vi "Front End.vi"() -> ()   [LabVIEW 2014]
uses:
  <vilib>/Utility/file.llb/Write To Spreadsheet File (DBL).vi
  <vilib>/Utility/file.llb/Write To Spreadsheet File (string).vi
  <vilib>/Utility/file.llb/Read From Spreadsheet File (DBL).vi
panel:
  in  "WebBrowser":refnum<k7>(container)
  in  "Tab Control":enum32{"Display", "Config"}(tab)
  in  "Control":enum32{"Auto", "Manual"}(tab)
  in  "Auto Stop":bool
  in  "Manual Stop":bool
  in  "Record Button":bool
  in  "Manual Throttle":dbl
  out "RPM":dbl
  out "Battery Life (h)":dbl
  out "Torque":dbl
  out "Horsepower":dbl
  in  "Main Stop":bool
  out "Flowrate":dbl
  out "Total Fuel":dbl
  out "Total Fuel Graph":cluster{u32, dbl}[](graph)
  out "Throttle":dbl
  in  "Time Unit":u16(ring)=1 items=["ms", "s"]
  in  "Control File":path
  in  "DAQ Device Name":tag="cDAQ1Mod1"
  in  "Output Directory":path
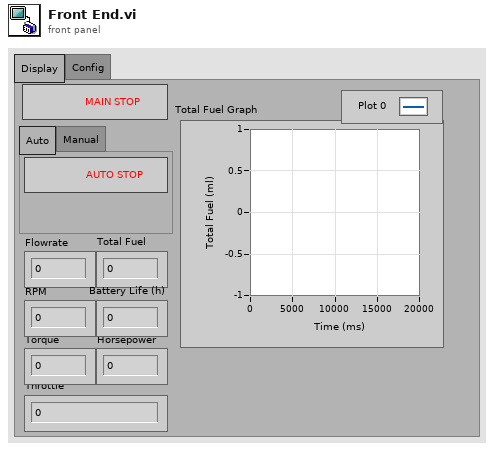
[diagram p1: front panel]
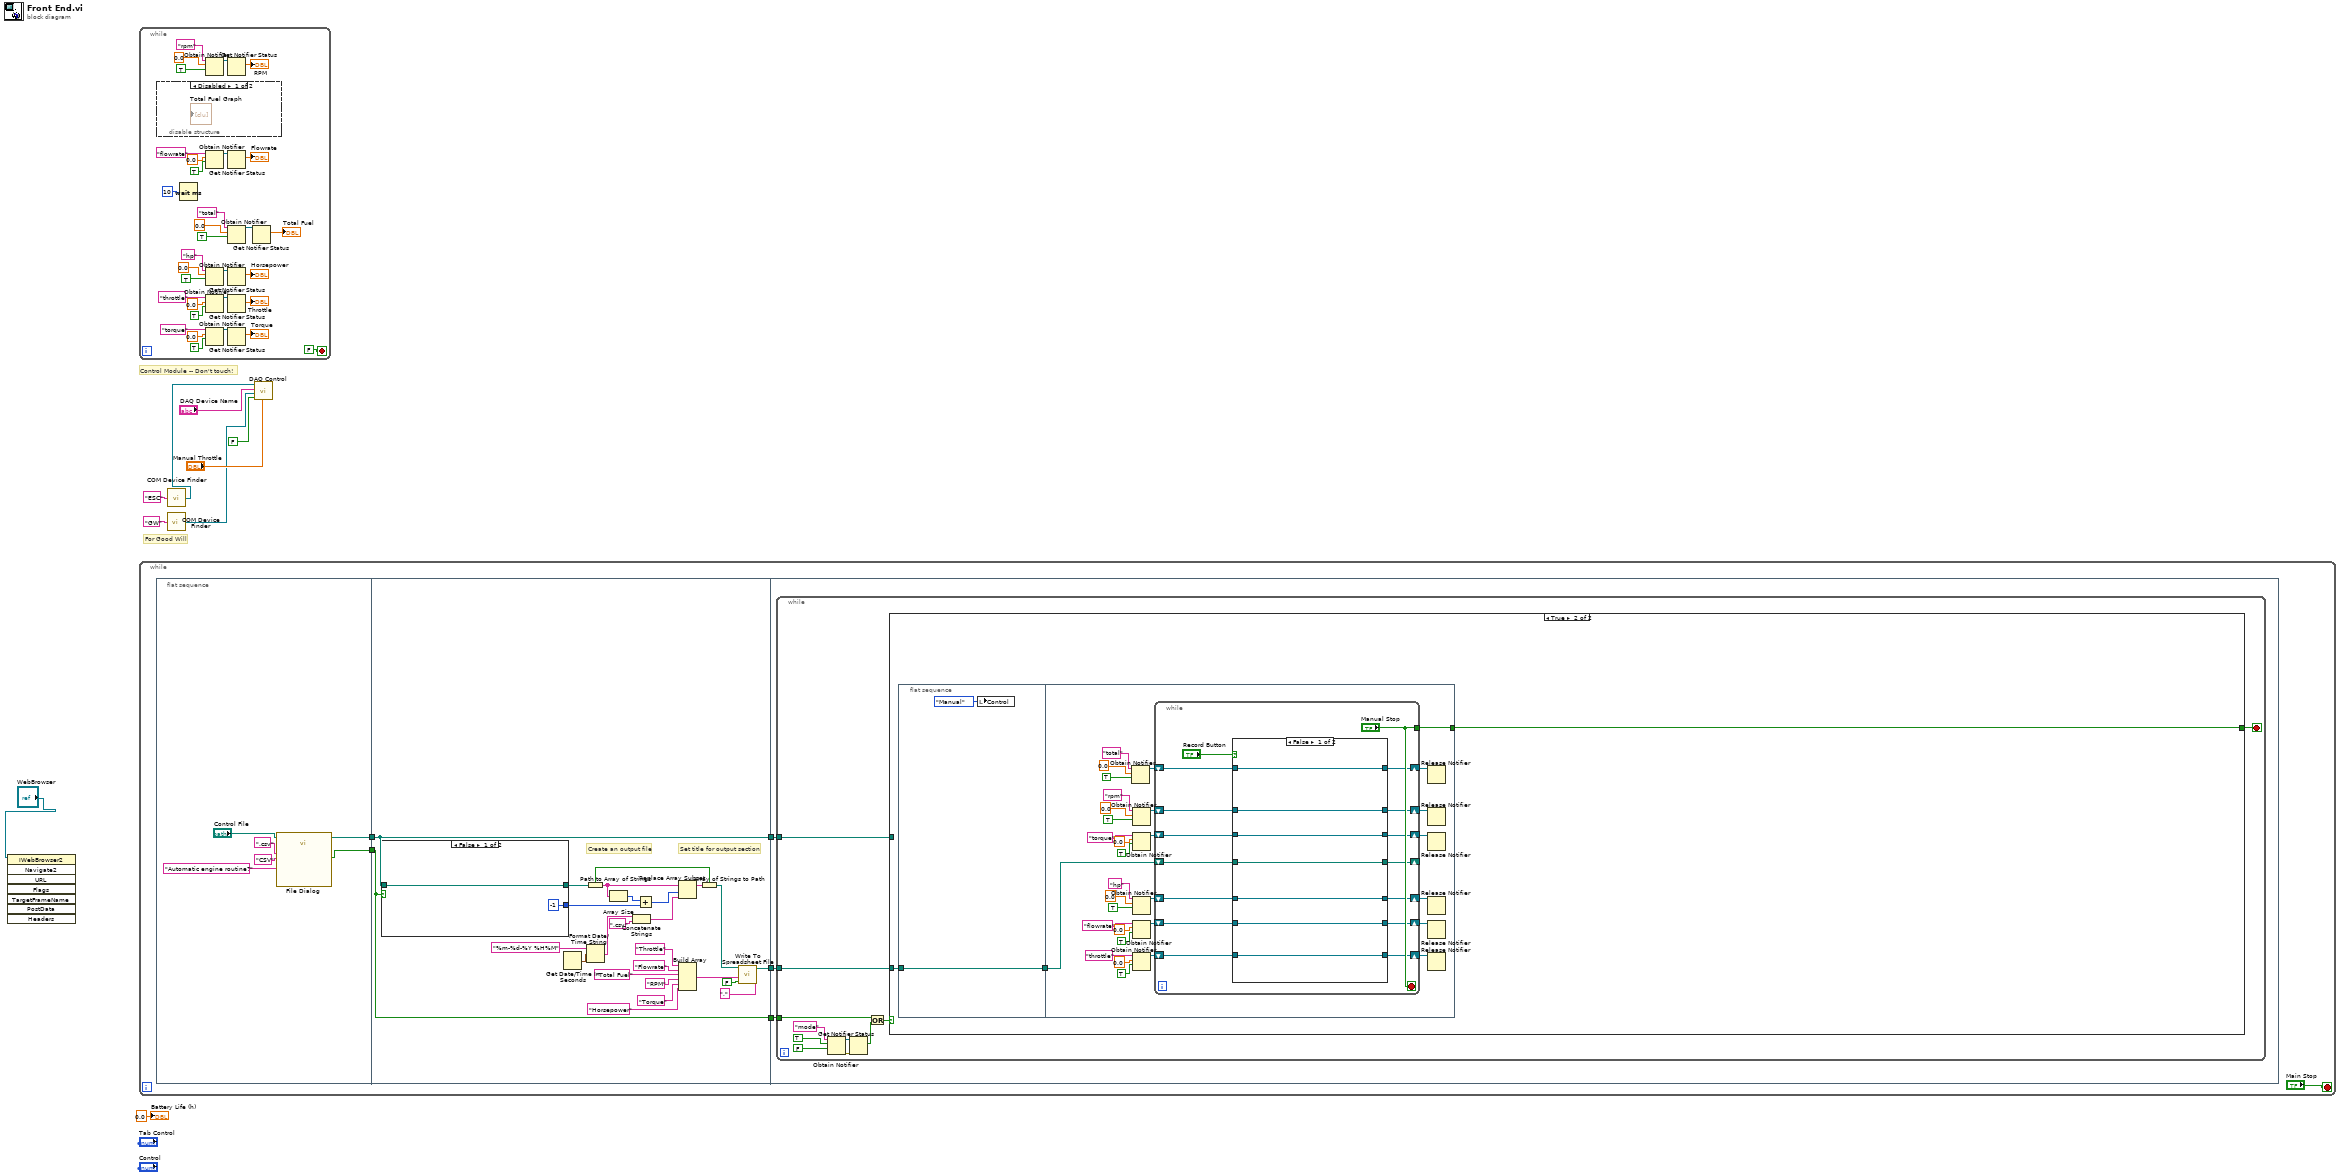
[diagram p0: block diagram]
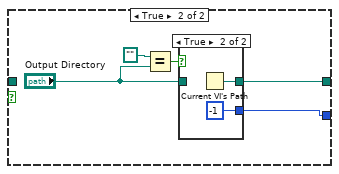
[diagram p3: hidden frame]
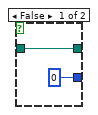
[diagram p4: hidden frame]
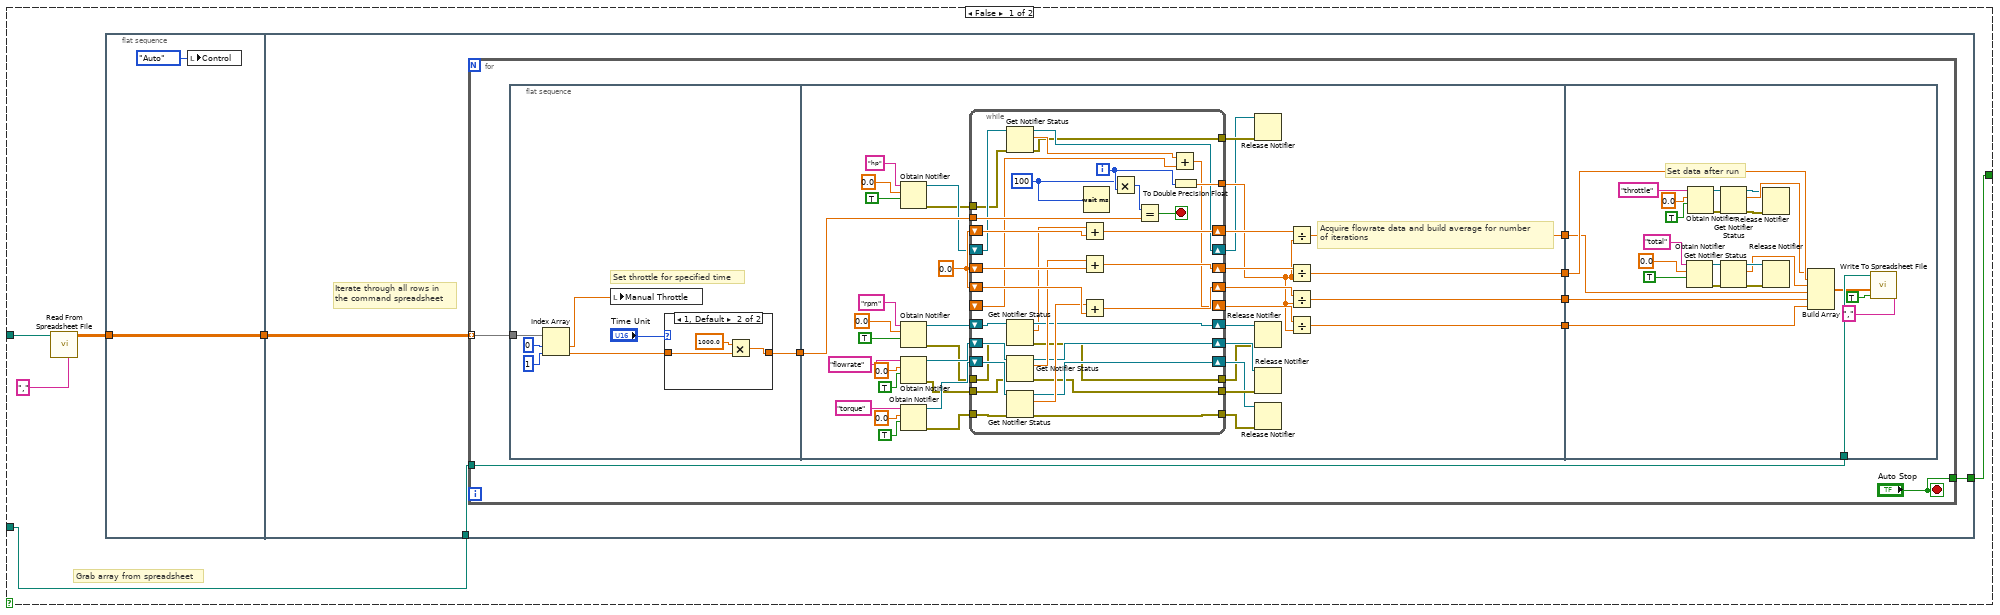
[diagram p5: hidden frame]
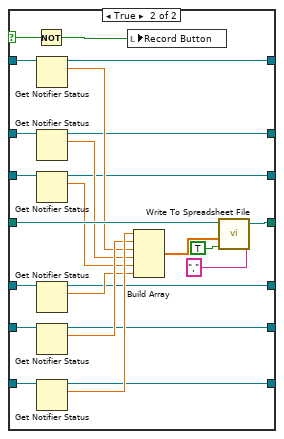
[diagram p7: hidden frame]
diagram:
  # "For Good Will"
  # "Control Module -- Don't touch!"
  n1 = invoke class="IWebBrowser2" method="Navigate2"(reference="WebBrowser") -> ()  [unwired: 7 in, 8 out]
  n2 = while {
    stop <- FALSE stop-if-true
    n3 = disable-structure shown="Disabled" {
      frame Disabled {
      }
      frame Enabled {
      }
    }
    n4 = Wait (ms)(milliseconds to wait=u32 10) -> ()  [unwired: 1 out]
    n5 = Obtain Notifier(name (unnamed)="rpm", notification data type=0.0, create if not found? (T)=TRUE) -> (notifier out=w21:refnum<notifier>)  [unwired: 1 in, 2 out]
    n6 = Obtain Notifier(name (unnamed)="flowrate", notification data type=0.0, create if not found? (T)=TRUE) -> (notifier out=w19:refnum<notifier>)  [unwired: 1 in, 2 out]
    n7 = Obtain Notifier(name (unnamed)="hp", notification data type=0.0, create if not found? (T)=TRUE) -> (notifier out=w20:refnum<notifier>)  [unwired: 1 in, 2 out]
    n8 = Obtain Notifier(name (unnamed)="throttle", notification data type=0.0, create if not found? (T)=TRUE) -> (notifier out=w18:refnum<notifier>)  [unwired: 1 in, 2 out]
    n9 = Obtain Notifier(name (unnamed)="torque", notification data type=0.0, create if not found? (T)=TRUE) -> (notifier out=w23:refnum<notifier>)  [unwired: 1 in, 2 out]
    n10 = Obtain Notifier(name (unnamed)="total", notification data type=0.0, create if not found? (T)=TRUE) -> (notifier out=w22:refnum<notifier>)  [unwired: 1 in, 2 out]
    n11 = Get Notifier Status(notifier=w21) -> (current notification=→"RPM":dbl)  [unwired: 1 in, 4 out]
    n12 = Get Notifier Status(notifier=w19) -> (current notification=→"Flowrate":dbl)  [unwired: 1 in, 4 out]
    n13 = Get Notifier Status(notifier=w20) -> (current notification=→"Horsepower":dbl)  [unwired: 1 in, 4 out]
    n14 = Get Notifier Status(notifier=w18) -> (current notification=→"Throttle":dbl)  [unwired: 1 in, 4 out]
    n15 = Get Notifier Status(notifier=w23) -> (current notification=→"Torque":dbl)  [unwired: 1 in, 4 out]
    n16 = Get Notifier Status(notifier=w22) -> (current notification=→"Total Fuel":dbl)  [unwired: 1 in, 4 out]
  }
  n17 = while {
    stop <- "Main Stop" stop-if-true
    n18 = flat-sequence {
      tunnel: [w53] -> w47
      tunnel: [w51] -> w46
      tunnel: [w72] -> w45
      tunnel: [w59] -> w44
      tunnel: w47 -> [w59]
      tunnel: [w56] -> w43
      tunnel: w46 -> [w56]
      tunnel: w45 -> [w92]
      tunnel: w44 -> [w91]
      tunnel: w43 -> [w90]
      frame #0 {
        n19 = call "File Dialog"("start path"="Control File", "prompt"="Automatic engine routine?", "pattern (all files)"=".csv", "pattern label"="CSV") -> ("selected path"=w53:path, "cancelled"=w51:bool)  [unwired: 8 in, 2 out]
      }
      frame #1 {
        # "Create an output file"
        # "Set title for output section"
        n20 = case shown="False" w56 {
          tunnel: w59 -> [w80 _]
          tunnel: [w80 w85] -> w58
          tunnel: [-1 w81] -> w54
          frame False {
          }
          frame True {
            n21 = Equal?(x=path "", y="Output Directory") -> (x = y?=w84:bool)
            n22 = case shown="True" w84 {
              tunnel: [w87 w89] -> w85
              tunnel: "Output Directory" -> [w87 _]
              tunnel: [0 -1] -> w81
              frame False {
              }
              frame True {
                n23 = Current VI's Path() -> (path=w89:path)
              }
            }
          }
        }
        n24 = Get Date/Time In Seconds() -> (seconds since 1Jan1904=w69:timestamp)
        n25 = Path to Array of Strings(0:w58) -> (1:w64:bool, 2:w71:string[])
        n26 = Format Date/Time String(time format string (%c)="%m-%d-%Y %H%M", seconds (now)=w69) -> (date/time string=w68:string)  [unwired: 1 in]
        n27 = Array Size(array=w71) -> (size(s)=w55:i32)
        n28 = Concatenate Strings(w68, ".csv") -> (w66:string)
        n29 = Add(x=w55, y=w54) -> (x+y=w70:i32)
        n30 = Replace Array Subset(array=w71, new element=w66, index=w70) -> (w65:string[])
        n31 = Build Array("Throttle" ("element"), "Flowrate", "Total Fuel" ("element"), "RPM" ("element"), "Torque" ("element"), "Horsepower" ("element")) -> (w74:string[])
        n32 = Array of Strings to Path(0:w65, 1:w64) -> (2:w63:path)
        n33 = call-poly <vilib>:"Write To Spreadsheet File.vi"("delimiter (\\t)"="," ("delimiter (\\t)"), "append to file? (new file:F)"=FALSE, "1D data"=w74, "file path (dialog if empty)"=w63) -> ("new file path (Not A Path if cancelled)"=w72:path)  [unwired: 4 in]
      }
      frame #2 {
        n34 = while {
          tunnel: w92 -> [w103]
          tunnel: w91 -> [w102]
          tunnel: w90 -> [w95]
          stop <- w93 stop-if-true
          n35 = Obtain Notifier(name (unnamed)="mode", notification data type=TRUE, create if not found? (T)=FALSE) -> (notifier out=w101:refnum<notifier>, error out=w98:errorcluster)  [unwired: 1 in, 1 out]
          n36 = Get Notifier Status(notifier=w101, error in (no error)=w98) -> (current notification=w96:bool)  [unwired: 4 out]
          n37 = Or(x=w95, y=w96) -> (x .or. y?=w94:bool)
          n38 = case shown="True" w94 {
            tunnel: w103 -> [w107 w233]
            tunnel: w102 -> [w106 _]
            tunnel: [w104 w231] -> w93
            frame False {
              # "Grab array from spreadsheet"
              n39 = call-poly <vilib>:"Read From Spreadsheet File.vi"("delimiter (\\t)"="," ("delimiter (\\t)"), "file path (dialog if empty)"=w106) -> ("all rows"=w109:dbl[][])  [unwired: 5 in, 4 out]
              n40 = flat-sequence {
                tunnel: w109 -> [w111]
                tunnel: [w111] -> w105
                tunnel: w107 -> [w113]
                tunnel: w105 -> [w114]
                tunnel: [w112] -> w104
                frame #0 {
                  n41 = local write "Control"(enum32{"Auto", "Manual"}."Auto" ("Control")) -> ()
                }
                frame #1 {
                  # "Iterate through all rows in \nthe command spreadsheet"
                  n42 = for {
                    tunnel: w114 -> [w122] mode=indexing
                    tunnel: w113 -> [w120]
                    tunnel: ["Auto Stop"] -> w112
                    stop <- "Auto Stop" stop-if-true
                    n43 = flat-sequence {
                      tunnel: w122 -> [w129]
                      tunnel: [w124] -> w121
                      tunnel: w121 -> [w172]
                      tunnel: [w165] -> w119
                      tunnel: [w164] -> w118
                      tunnel: [w163] -> w117
                      tunnel: [w162] -> w116
                      tunnel: w120 -> [w229]
                      tunnel: w119 -> [w227]
                      tunnel: w118 -> [w226]
                      tunnel: w117 -> [w225]
                      tunnel: w116 -> [w224]
                      frame #0 {
                        # "Set throttle for specified time"
                        n44 = Index Array(array=w129, index #1=0 ("index"), index #2=1 ("index")) -> (element #1=w123:dbl, element #2=w125:dbl)
                        n45 = local write "Manual Throttle"(w123) -> ()
                        n46 = case shown="1, Default" "Time Unit" {
                          tunnel: w125 -> [w130 w133]
                          tunnel: [w130 w131] -> w124
                          frame 0 {
                          }
                          frame 1, Default {
                            n47 = Multiply(x=1000.0, y=w133) -> (x*y=w131:dbl)
                          }
                        }
                      }
                      frame #1 {
                        w171 = 0.0
                        # "Acquire flowrate data and build average for number\nof iterations"
                        n48 = Obtain Notifier(name (unnamed)="hp", notification data type=0.0, create if not found? (T)=TRUE) -> (notifier out=w149:refnum<notifier>, error out=w136:errorcluster)  [unwired: 1 in, 1 out]
                        n49 = Obtain Notifier(name (unnamed)="rpm", notification data type=0.0, create if not found? (T)=TRUE) -> (notifier out=w146:refnum<notifier>, error out=w137:errorcluster)  [unwired: 1 in, 1 out]
                        n50 = Obtain Notifier(name (unnamed)="flowrate", notification data type=0.0, create if not found? (T)=TRUE) -> (notifier out=w148:refnum<notifier>, error out=w144:errorcluster)  [unwired: 1 in, 1 out]
                        n51 = Obtain Notifier(name (unnamed)="torque", notification data type=0.0, create if not found? (T)=TRUE) -> (notifier out=w147:refnum<notifier>, error out=w140:errorcluster)  [unwired: 1 in, 1 out]
                        n52 = while {
                          shift-right: [w195] -> w167
                          shift-left: w171 -> [w196]
                          tunnel: w172 -> [w206]
                          tunnel: [w201] -> w166
                          shift-right: [w199] -> w170
                          shift-left: w171 -> [w200]
                          shift-right: [w197] -> w169
                          shift-left: w171 -> [w198]
                          shift-right: [w194] -> w168
                          shift-left: _ -> [w193]
                          shift-right: [w190] -> w134
                          shift-left: w149 -> [w191]
                          shift-right: [w185] -> w145
                          shift-left: w148 -> [w189]
                          shift-right: [w184] -> w142
                          shift-left: w147 -> [w187]
                          shift-right: [w182] -> w139
                          shift-left: w146 -> [w183]
                          tunnel: w144 -> [w180]
                          tunnel: [w179] -> w143
                          tunnel: [w178] -> w141
                          tunnel: w140 -> [w177]
                          tunnel: [w176] -> w138
                          tunnel: w137 -> [w175]
                          tunnel: w136 -> [w174]
                          tunnel: [w173] -> w135
                          i -> [w204]
                          stop <- w205 stop-if-true
                          w203 = u32 100 ("milliseconds to wait")
                          n53 = Get Notifier Status(notifier=w191, error in (no error)=w174) -> (notifier out=w190:refnum<notifier>, current notification=w192:dbl, error out=w173:errorcluster)  [unwired: 2 out]
                          n54 = Get Notifier Status(notifier=w183, error in (no error)=w175) -> (notifier out=w182:refnum<notifier>, current notification=w181:dbl, error out=w176:errorcluster)  [unwired: 2 out]
                          n55 = Get Notifier Status(notifier=w189, error in (no error)=w180) -> (notifier out=w185:refnum<notifier>, current notification=w188:dbl, error out=w179:errorcluster)  [unwired: 2 out]
                          n56 = Get Notifier Status(notifier=w187, error in (no error)=w177) -> (notifier out=w184:refnum<notifier>, current notification=w186:dbl, error out=w178:errorcluster)  [unwired: 2 out]
                          n57 = Add(x=w181, y=w198) -> (x+y=w197:dbl)
                          n58 = Add(x=w188, y=w200) -> (x+y=w199:dbl)
                          n59 = Add(x=w186, y=w196) -> (x+y=w195:dbl)
                          n60 = Wait (ms)(milliseconds to wait=w203) -> ()  [unwired: 1 out]
                          n61 = Multiply(x=w203, y=w204) -> (x*y=w202:u32)
                          n62 = Equal?(x=w202, y=w206) -> (x = y?=w205:bool)
                          n63 = Add(x=w192, y=w193) -> (x+y=w194:dbl)
                          n64 = To Double Precision Float(number=w204) -> (double precision float=w201:dbl)
                        }
                        n65 = Release Notifier(notifier=w134, error in (no error)=w135) -> ()  [unwired: 1 in, 3 out]
                        n66 = Release Notifier(notifier=w139, error in (no error)=w138) -> ()  [unwired: 1 in, 3 out]
                        n67 = Release Notifier(notifier=w145, error in (no error)=w143) -> ()  [unwired: 1 in, 3 out]
                        n68 = Release Notifier(notifier=w142, error in (no error)=w141) -> ()  [unwired: 1 in, 3 out]
                        n69 = Divide(x=w169, y=w166) -> (x/y=w164:dbl)
                        n70 = Divide(x=w170, y=w166) -> (x/y=w165:dbl)
                        n71 = Divide(x=w167, y=w166) -> (x/y=w163:dbl)
                        n72 = Divide(x=w168, y=w166) -> (x/y=w162:dbl)
                      }
                      frame #2 {
                        # "Set data after run"
                        n73 = Obtain Notifier(name (unnamed)="total", notification data type=0.0, create if not found? (T)=TRUE) -> (notifier out=w214:refnum<notifier>, error out=w209:errorcluster)  [unwired: 1 in, 1 out]
                        n74 = Obtain Notifier(name (unnamed)="throttle", notification data type=0.0, create if not found? (T)=TRUE) -> (notifier out=w222:refnum<notifier>, error out=w216:errorcluster)  [unwired: 1 in, 1 out]
                        n75 = Get Notifier Status(notifier=w222, error in (no error)=w216) -> (notifier out=w217:refnum<notifier>, current notification=w218:dbl, error out=w215:errorcluster)  [unwired: 2 out]
                        n76 = Get Notifier Status(notifier=w214, error in (no error)=w209) -> (notifier out=w210:refnum<notifier>, current notification=w207:dbl, error out=w208:errorcluster)  [unwired: 2 out]
                        n77 = Release Notifier(notifier=w217, error in (no error)=w215) -> ()  [unwired: 1 in, 3 out]
                        n78 = Release Notifier(notifier=w210, error in (no error)=w208) -> ()  [unwired: 1 in, 3 out]
                        n79 = Build Array(w218, w227, w207, w226, w225, w224) -> (w223:dbl[])
                        n80 = call-poly <vilib>:"Write To Spreadsheet File.vi"("delimiter (\\t)"="," ("delimiter (\\t)"), "append to file? (new file:F)"=TRUE, "1D data"=w223, "file path (dialog if empty)"=w229) -> ()  [unwired: 4 in, 1 out]
                      }
                    }
                  }
                }
              }
            }
            frame True {
              n81 = flat-sequence {
                tunnel: w233 -> [w235]
                tunnel: [w235] -> w232
                tunnel: w232 -> [w267]
                tunnel: [w266] -> w231
                frame #0 {
                  n82 = local write "Control"(enum32{"Auto", "Manual"}."Manual" ("Tab Control 2")) -> ()
                }
                frame #1 {
                  n83 = Obtain Notifier(name (unnamed)="total", notification data type=0.0, create if not found? (T)=TRUE) -> (notifier out=w245:refnum<notifier>)  [unwired: 1 in, 2 out]
                  n84 = Obtain Notifier(name (unnamed)="rpm", notification data type=0.0, create if not found? (T)=TRUE) -> (notifier out=w244:refnum<notifier>)  [unwired: 1 in, 2 out]
                  n85 = Obtain Notifier(name (unnamed)="torque", notification data type=0.0, create if not found? (T)=TRUE) -> (notifier out=w243:refnum<notifier>)  [unwired: 1 in, 2 out]
                  n86 = Obtain Notifier(name (unnamed)="hp", notification data type=0.0, create if not found? (T)=TRUE) -> (notifier out=w242:refnum<notifier>)  [unwired: 1 in, 2 out]
                  n87 = Obtain Notifier(name (unnamed)="flowrate", notification data type=0.0, create if not found? (T)=TRUE) -> (notifier out=w246:refnum<notifier>)  [unwired: 1 in, 2 out]
                  n88 = Obtain Notifier(name (unnamed)="throttle", notification data type=0.0, create if not found? (T)=TRUE) -> (notifier out=w247:refnum<notifier>)  [unwired: 1 in, 2 out]
                  n89 = while {
                    tunnel: ["Manual Stop"] -> w266
                    shift-right: [w268] -> _
                    shift-left: w267 -> [w282]
                    shift-right: [w270] -> w237
                    shift-left: w246 -> [w279]
                    shift-right: [w273] -> w240
                    shift-left: w245 -> [w278]
                    shift-right: [w269] -> w236
                    shift-left: w247 -> [w280]
                    shift-right: [w274] -> w241
                    shift-left: w243 -> [w276]
                    shift-right: [w272] -> w239
                    shift-left: w244 -> [w277]
                    shift-right: [w271] -> w238
                    shift-left: w242 -> [w275]
                    stop <- "Manual Stop" stop-if-true
                    n90 = case shown="False" "Record Button" {
                      selector: "Record Button" -> [_ w315]
                      tunnel: w282 -> [w284 w313]
                      tunnel: w280 -> [w285 w309]
                      tunnel: w279 -> [w286 w307]
                      tunnel: w278 -> [w289 w305]
                      tunnel: w277 -> [w288 w303]
                      tunnel: w276 -> [w290 w301]
                      tunnel: w275 -> [w287 w299]
                      tunnel: [w290 w297] -> w274
                      tunnel: [w289 w296] -> w273
                      tunnel: [w288 w295] -> w272
                      tunnel: [w287 w294] -> w271
                      tunnel: [w286 w293] -> w270
                      tunnel: [w285 w292] -> w269
                      tunnel: [w284 w291] -> w268
                      frame False {
                      }
                      frame True {
                        n91 = Not(x=w315) -> (.not. x?=w314:bool)
                        n92 = Get Notifier Status(notifier=w305) -> (notifier out=w296:refnum<notifier>, current notification=w304:dbl)  [unwired: 1 in, 3 out]
                        n93 = Get Notifier Status(notifier=w303) -> (notifier out=w295:refnum<notifier>, current notification=w302:dbl)  [unwired: 1 in, 3 out]
                        n94 = Get Notifier Status(notifier=w301) -> (notifier out=w297:refnum<notifier>, current notification=w300:dbl)  [unwired: 1 in, 3 out]
                        n95 = Get Notifier Status(notifier=w299) -> (notifier out=w294:refnum<notifier>, current notification=w298:dbl)  [unwired: 1 in, 3 out]
                        n96 = Get Notifier Status(notifier=w307) -> (notifier out=w293:refnum<notifier>, current notification=w306:dbl)  [unwired: 1 in, 3 out]
                        n97 = Get Notifier Status(notifier=w309) -> (notifier out=w292:refnum<notifier>, current notification=w308:dbl)  [unwired: 1 in, 3 out]
                        n98 = local write "Record Button"(w314) -> ()
                        n99 = Build Array(w308, w306, w304, w302, w300, w298) -> (w312:dbl[])
                        n100 = call-poly <vilib>:"Write To Spreadsheet File.vi"("delimiter (\\t)"="," ("delimiter (\\t)"), "append to file? (new file:F)"=TRUE, "1D data"=w312, "file path (dialog if empty)"=w313) -> ("new file path (Not A Path if cancelled)"=w291:path)  [unwired: 4 in]
                      }
                    }
                  }
                  n101 = Release Notifier(notifier=w240) -> ()  [unwired: 2 in, 3 out]
                  n102 = Release Notifier(notifier=w239) -> ()  [unwired: 2 in, 3 out]
                  n103 = Release Notifier(notifier=w241) -> ()  [unwired: 2 in, 3 out]
                  n104 = Release Notifier(notifier=w238) -> ()  [unwired: 2 in, 3 out]
                  n105 = Release Notifier(notifier=w237) -> ()  [unwired: 2 in, 3 out]
                  n106 = Release Notifier(notifier=w236) -> ()  [unwired: 2 in, 3 out]
                }
              }
            }
          }
        }
      }
    }
  }
  n107 = call "COM Device Finder.vi"("*IDN?"="GW") -> ("VISA resource name"=w2:refnum<visa-resource-name>)
  n108 = call "COM Device Finder.vi"("*IDN?"="ESC") -> ("VISA resource name"=w3:refnum<visa-resource-name>)
  n109 = call "DAQ Control.vi"("Throttle"="Manual Throttle", 8:FALSE, "PSU VISA"=w2, "DAQ Device Name"="DAQ Device Name", "Fuelflow VISA"=w3) -> ()  [unwired: 3 in, 4 out]
  "Battery Life (h)" <- 0.0 ("Battery Life (h)")
